vi "calculateNewPhase.vi"(8 "error in (no error)":errorcluster, 11 "SingleToneAction in":refnum<class "SingleToneAction.lvclass">) -> (0 "error out":errorcluster, 3 "SingleToneAction out":refnum<class "SingleToneAction.lvclass">)   [LabVIEW 2009, in "Views.lvlib" / "ScriptEditor.lvlib" / "SingleToneAction.lvclass"]
uses:
  SingleToneAction.lvclass
  Tools/Scripting/ScriptingEvent/ScriptEvents/SingleTone/SingleTone.lvclass
  Tools/Scripting/ScriptingEvent/ScriptEvents/SingleToneArray/SingleToneArray.lvclass
  SingleToneAction.lvclass/SingleToneAction.ctl
  Tools/Scripting/ScriptingEvent/ScriptEvent.lvclass
  Tools/DatabaseHelpers/Database Objects/Channel/Channel.lvclass
  ActionPanel.lvclass
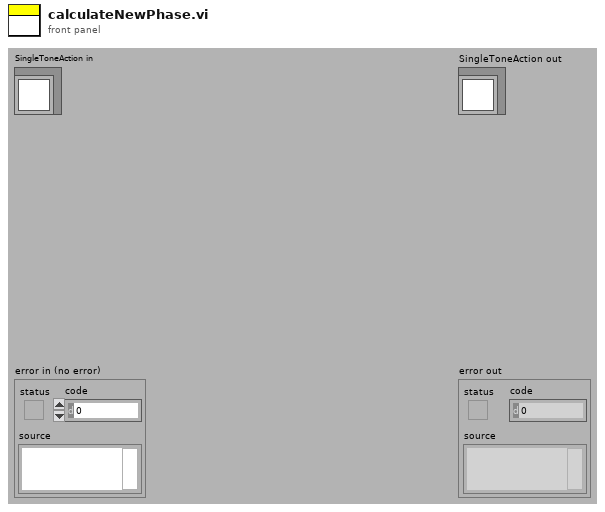
[diagram p1: front panel]
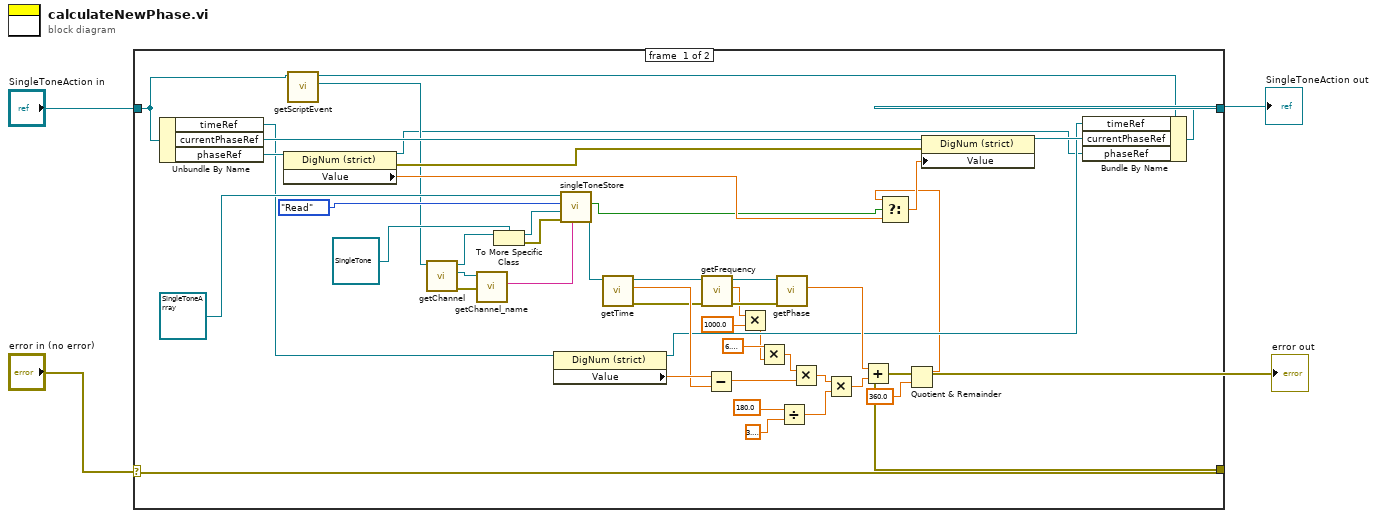
[diagram p0: block diagram]
diagram:
  n1 = case shown="No Error" "error in (no error)" {
    selector: "error in (no error)" -> [w50 w52]
    tunnel: [w50 w52] -> w3
    tunnel: [w10 w51] -> w1
    tunnel: "SingleToneAction in" -> [w39 w51]
    frame #0 {
      n2 = Unbundle By Name(w39) -> ("timeRef"=w32:refnum<vi>, "currentPhaseRef"=w49:refnum<vi>, "phaseRef"=w47:refnum<vi>)
      n3 = property class="DigNum (strict)"(reference=w47) -> (reference out=w11:refnum<vi>, error out=w48:errorcluster, "Value"=w45:dbl)  [unwired: 1 in]
      n4 = call "getScriptEvent.vi"("ActionPanel.lvclass in"=w39) -> ("ScriptEvent.lvclass"=w34:refnum<class "ScriptEvent.lvclass">, "ActionPanel.lvclass out"=w14:refnum<class "SingleToneAction.lvclass">)  [unwired: 8 in, 1 out]
      n5 = call-dynamic "getChannel.vi"("ScriptEvent.lvclass in"=w34) -> ("error out"=w40:errorcluster, "Channel.lvclass"=w41:refnum<class "Channel.lvclass">, "ScriptEvent.lvclass out"=w33:refnum<class "ScriptEvent.lvclass">)  [unwired: 8 in]
      n6 = call "getChannel_name.vi"("error in (no error)"=w40, "Channel.lvclass in"=w41) -> ("channel_name"=w38:string)  [unwired: 7 in, 2 out]
      n7 = To More Specific Class(target class=refnum<class "SingleTone.lvclass"> refnum ("Tools.lvlib:Scripting.lvlib:SingleTone.lvclass"), reference=w33) -> (specific class reference=w35:refnum<class "SingleTone.lvclass">, error out=w37:errorcluster)  [unwired: 1 in]
      n8 = property class="DigNum (strict)"(reference=w32) -> (reference out=w12:refnum<vi>, "Value"=w30:dbl)  [unwired: 1 in, 1 out]
      n9 = call "singleToneStore.vi"("channel_name"=w38, "error in (no error)"=w37, "SingleTone.lvclass"=w35, "action"=enum16{"Write", "Read"}."Read", "SingleToneArray in"=refnum<class "SingleToneArray.lvclass"> refnum) -> ("SingleTone.lvclass out"=w31:refnum<class "SingleTone.lvclass">, "found?"=w44:bool)  [unwired: 3 in, 2 out]
      n10 = call "getTime.vi"("ScriptEvent.lvclass in"=w31) -> ("error out"=w27:errorcluster, "time"=w29:dbl, "ScriptEvent.lvclass out"=w28:refnum<class "SingleTone.lvclass">)  [unwired: 8 in]
      n11 = call "getFrequency.vi"("error in (no error)"=w27, "SingleTone.lvclass in"=w28) -> ("error out"=w25:errorcluster, "frequency"=w7:dbl, "SingleTone.lvclass out"=w26:refnum<class "SingleTone.lvclass">)  [unwired: 7 in]
      n12 = Subtract(x=w30, y=w29) -> (x-y=w23:dbl)
      n13 = Multiply(x=w7, y=1000.0) -> (x*y=w5:dbl)
      n14 = Multiply(x=6.283185307179586, y=w5) -> (x*y=w24:dbl)
      n15 = call "getPhase.vi"("error in (no error)"=w25, "SingleTone.lvclass in"=w26) -> ("phase"=w17:dbl)  [unwired: 7 in, 2 out]
      n16 = Divide(x=180.0, y=3.141592653589793) -> (x/y=w19:dbl)
      n17 = Multiply(x=w24, y=w23) -> (x*y=w20:dbl)
      n18 = Multiply(x=w20, y=w19) -> (x*y=w18:dbl)
      n19 = Add(x=w17, y=w18) -> (x+y=w16:dbl)
      n20 = Quotient & Remainder(x=w16, y=360.0) -> (x-y*floor(x/y)=w9:dbl)  [unwired: 1 out]
      n21 = Select(t=w9, s=w44, f=w45) -> (s? t:f=w46:dbl)
      n22 = property class="DigNum (strict)"(reference=w49, error in=w48, "Value"=w46) -> (reference out=w13:refnum<vi>)  [unwired: 1 out]
      n23 = Bundle By Name(cluster=w14, "timeRef"=w12, "currentPhaseRef"=w13, "phaseRef"=w11) -> (w10:refnum<class "SingleToneAction.lvclass">)
    }
    frame #1 {
    }
  }
  "error out" <- w3
  "SingleToneAction out" <- w1
